vi "Get_STREAM_TYPE.vi"(5 "Device Number":T2, 7 "Update":bool, 11 "Protocol (in)":T1=enum."SPI") -> (3 "Protocol (out)":T1=enum."SPI")   [LabVIEW 2025]
uses:
  _TypeDefs/FRIC_navX_DeviceNumbersTypeDef.ctl
  _TypeDefs/Z900_navX_ProtocolTypeDef.ctl
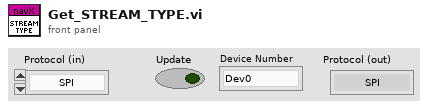
[diagram p1: front panel]
types:
  T1 = typedef "Z900_navX_ProtocolTypeDef.ctl" = enum16{"SERIAL", "I2C", "SPI"}
  T2 = typedef "FRIC_navX_DeviceNumbersTypeDef.ctl" = enum16{"Dev0", "Dev1", "Dev2", "Dev3"}
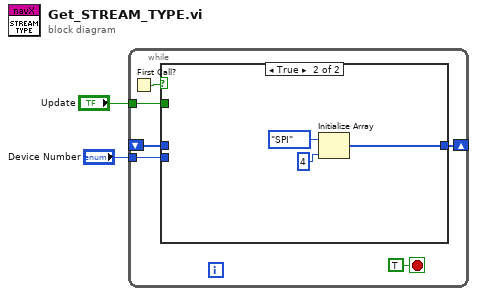
[diagram p0: block diagram]
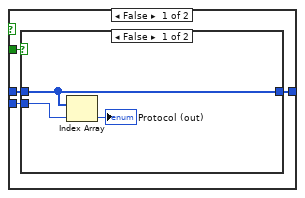
[diagram p2: hidden frame]
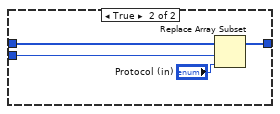
[diagram p3: hidden frame]
diagram:
  n1 = while {
    shift-right: [w8] -> _
    shift-left: _ -> [w5]
    tunnel: "Update" -> [w6]
    tunnel: "Device Number" -> [w4]
    stop <- TRUE stop-if-true
    n2 = First Call?() -> (First Call?: T/F=w3:bool)
    n3 = case shown="True" w3 {
      tunnel: [w12 w22] -> w8
      tunnel: w6 -> [w11 _]
      tunnel: w5 -> [w10 _]
      tunnel: w4 -> [w9 _]
      frame False {
        n4 = case shown="False" w11 {
          tunnel: [w15 w18] -> w12
          tunnel: w10 -> [w15 w19]
          tunnel: w9 -> [w14 w17]
          frame False {
            n5 = Index Array(array=w15, index=w14) -> (element=→"Protocol (out)":T1)
          }
          frame True {
            n6 = Replace Array Subset(array=w19, new element="Protocol (in)", index=w17) -> (w18:T1[])
          }
        }
      }
      frame True {
        n7 = Initialize Array(Z900_navX_ProtocolTypeDef."SPI" ("Protocol (in)"), 4 ("dimension size")) -> (w22:T1[])
      }
    }
  }
